vi "Test CPC.vi"() -> ()   [LabVIEW 2014]
uses:
  CPC.lvclass
  3022A/Flow.ctl
panel:
  out "pumpV":dbl
  out "Ready?":bool
  out "cmdGood":bool
  in  "Flow Rate":T1
  out "Q":dbl
  out "instrT":cluster{"cond T":dbl, "sat T":dbl, "opt T":dbl}
  out "Conc":dbl
  out "error out":errorcluster
  in  "Boolean":bool
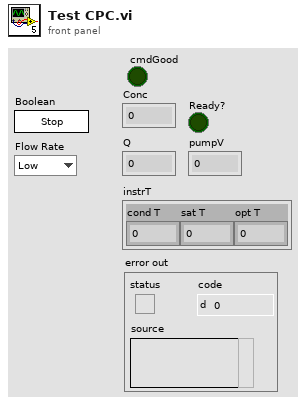
[diagram p1: front panel]
types:
  T1 = typedef "CPC.lvclass/Flow.ctl" = enum16{"Low", "High"}
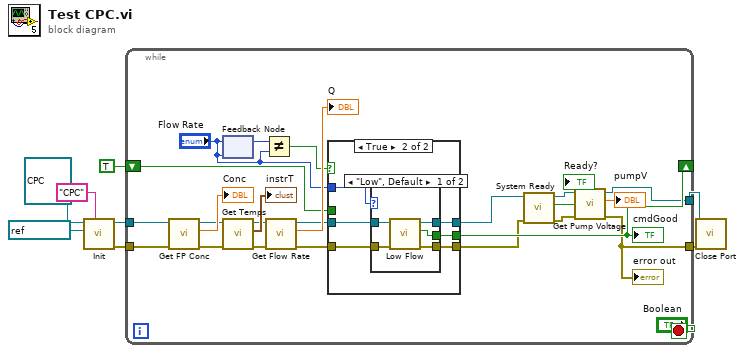
[diagram p0: block diagram]
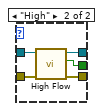
[diagram p3: hidden frame]
diagram:
  n1 = call-dynamic "Init.vi"("Name"="CPC", "Port"=refnum<visa-resource-name> "COM4", "CPC in"=refnum<class "CPC.lvclass"> refnum ("CPC.lvclass")) -> ("error out"=w6:errorcluster, "CPC out"=w5:refnum<class "CPC.lvclass">)  [unwired: 7 in]
  n2 = while {
    tunnel: w6 -> [w31]
    tunnel: w5 -> [w32]
    tunnel: [w10] -> w4
    tunnel: [w9] -> w3
    shift-right: [w18] -> _
    shift-left: TRUE ("cmdGood") -> [w17]
    stop <- "Boolean" stop-if-true
    n3 = call-dynamic "Get FP Conc.vi"("error in"=w31, "CPC in"=w32) -> ("error out"=w28:errorcluster, "Conc"=→"Conc":dbl, "CPC out"=w29:refnum<class "CPC.lvclass">)  [unwired: 7 in]
    n4 = feedback-in #1("Flow Rate") -> ()
    n5 = feedback #1("Flow Rate") -> (w21:T1)
    n6 = call-dynamic "Get Temps.vi"("error in"=w28, "CPC in"=w29) -> ("error out"=w25:errorcluster, "instrT"=→"instrT":cluster{"cond T":dbl, "sat T":dbl, "opt T":dbl}, "CPC out"=w26:refnum<class "CPC.lvclass">)  [unwired: 7 in]
    n7 = Not Equal?(x=w21, y="Flow Rate") -> (x != y?=w20:bool)
    n8 = call-dynamic "Get Flow Rate.vi"("error in"=w25, "CPC in"=w26) -> ("error out"=w22:errorcluster, "Q"=→"Q":dbl, "CPC out"=w23:refnum<class "CPC.lvclass">)  [unwired: 7 in]
    n9 = case shown="True" w20 {
      tunnel: w23 -> [w36 w42]
      tunnel: w22 -> [w35 w41]
      tunnel: "Flow Rate" -> [_ w40]
      tunnel: [w36 w39] -> w16
      tunnel: [w35 w38] -> w15
      tunnel: [w34 w37] -> w18
      tunnel: w17 -> [w34 _]
      frame False {
      }
      frame True {
        n10 = case shown="\"Low\", Default" w40 {
          tunnel: w42 -> [w47 w52]
          tunnel: w41 -> [w46 w51]
          tunnel: [w45 w49] -> w39
          tunnel: [w44 w50] -> w38
          tunnel: [w43 w48] -> w37
          frame "Low", Default {
            n11 = call-dynamic "Low Flow.vi"("error in"=w46, "CPC in"=w47) -> ("error out"=w44:errorcluster, "cmdGood"=w43:bool, "CPC out"=w45:refnum<class "CPC.lvclass">)  [unwired: 7 in]
          }
          frame "High" {
            n12 = call-dynamic "High Flow.vi"("error in"=w51, "CPC in"=w52) -> ("error out"=w50:errorcluster, "cmdGood"=w48:bool, "CPC out"=w49:refnum<class "CPC.lvclass">)  [unwired: 7 in]
          }
        }
      }
    }
    "cmdGood" <- w18
    n13 = call-dynamic "System Ready.vi"("error in"=w15, "CPC in"=w16) -> ("error out"=w13:errorcluster, "Ready?"=→"Ready?":bool, "CPC out"=w14:refnum<class "CPC.lvclass">)  [unwired: 7 in]
    n14 = call-dynamic "Get Pump Voltage.vi"("error in"=w13, "CPC in"=w14) -> ("error out"=w9:errorcluster, "pumpV"=→"pumpV":dbl, "CPC out"=w10:refnum<class "CPC.lvclass">)  [unwired: 7 in]
    "error out" <- w9
  }
  n15 = call-dynamic "Close Port.vi"("error in (no error)"=w3, "Serial IO in"=w4) -> ()  [unwired: 8 in, 2 out]
